vi "Odometry.vi"   [LabVIEW 2017]
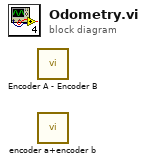
[diagram p0: block diagram]
diagram:
  n1 = call "Encoder A - Encoder B.vi"() -> ()  [unwired: 1 out]
  n2 = call "encoder a+encoder b.vi"() -> ()  [unwired: 12 in]
